vi "Marker Data.vi"(5 "Marker (1)":i32=1, 7 "Channel (1)":i32=1, 8 "error in (no error)":errorcluster, 11 "VISA resource name":refnum<visa-resource-name>) -> (0 "error out":errorcluster, 1 "Y Real Value":dbl format="%^.2e", 2 "X Value":dbl format="%^.2e", 3 "VISA resource name out":refnum<visa-resource-name>, 4 "Y Imaginary Value":dbl format="%^.2e")   [LabVIEW 2022 SP3, in "Agilent ENA Series.lvlib"]
doc: "Reads out the response value of selected marker, for the active trace of selected channel.\n\nNote:\nWhen the reference marker mode is enabled, the readout value is the value relative to the reference marker."
uses:
  Agilent ENA Series.lvlib
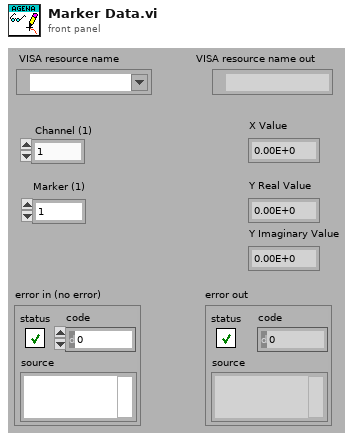
[diagram p1: front panel]
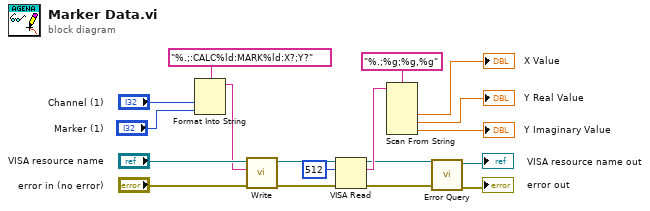
[diagram p0: block diagram]
diagram:
  n1 = Format Into String(format string="%.;:CALC%ld:MARK%ld:X?;Y?", "Channel (1)", "Marker (1)") -> (resulting string=w9:string)  [unwired: 2 in, 1 out]
  n2 = call "Write.vi"("error in (no error)"="error in (no error)", "String ()"=w9, "VISA resource name"="VISA resource name") -> ("error out"=w15:errorcluster, "VISA resource name out"=w16:refnum<visa-resource-name>)  [unwired: 6 in, 1 out]
  n3 = VISA Read(VISA resource name=w16, byte count=u32 512, error in (no error)=w15) -> (VISA resource name out=w4:refnum<visa-resource-name>, read buffer=w13:string, error out=w3:errorcluster)  [unwired: 1 out]
  n4 = Scan From String(format string="%.;%g;%g,%g", input string=w13) -> (output 1=→"X Value":dbl, output 2=→"Y Real Value":dbl, output 3=→"Y Imaginary Value":dbl)  [unwired: 5 in, 3 out]
  n5 = call "Error Query.vi"("error in (no error)"=w3, "VISA resource name"=w4) -> ("error out"=→"error out":errorcluster, "VISA resource name out"=→"VISA resource name out":refnum<visa-resource-name>)  [unwired: 6 in, 2 out]
